vi "Get Window Constants.vi"(11 "window info":T1={"window type"=10, "window length"=2048} {"window type" items=["None"=0, "Hanning"=1, "Hamming"=2, "Blackman-Harris"=3, "Exact Blackman"=4, "Blackman"=5, "Flat Top"=6, "4 Term B-Harris"=7, "7 Term B-Harris"=8, "Low Sidelobe"=9, "Gaussian"=62]; "window length" min=0}) -> (1 "multiply factor":dbl format="%.2f", 3 "window constants":cluster{"eq noise BW":dbl, "coherent gain":dbl} {"coherent gain" format="%.2f"; "eq noise BW" format="%.2f"})   [LabVIEW 2017, in "SoundVib_Gabor.lvlib"]
uses:
  <vilib>/addons/Sound and Vibration/Order Analysis/Gabor Order Tracking/SoundVib_Gabor.lvlib
  <vilib>/addons/Sound and Vibration/Order Analysis/Ref Gabor Order Tracking/window information.ctl
  <vilib>/Analysis/0measdsp.llb/Scaled Time Domain Window (DBL).vi
  <vilib>/Analysis/NI_AALPro.lvlib
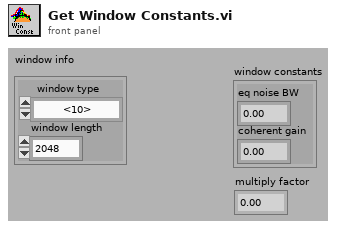
[diagram p1: front panel]
types:
  T1 = typedef "SoundVib_Gabor.lvlib/window information.ctl" = cluster{"window type":u32, "window length":i32}
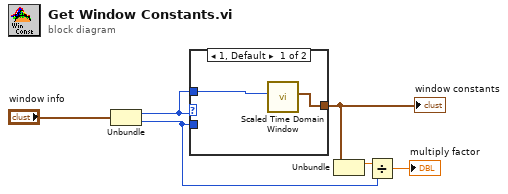
[diagram p0: block diagram]
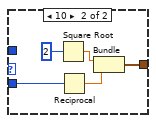
[diagram p2: hidden frame]
diagram:
  n1 = Unbundle("window info") -> ("window type"=w1:u32, "window length"=w3:i32)
  n2 = case shown="1, Default" w1 {
    tunnel: w3 -> [_ w13]
    tunnel: [w8 w9] -> w4
    tunnel: w1 -> [w7 _]
    frame 1, Default {
      n3 = call-poly <vilib>:"Scaled Time Domain Window.vi"("window"=w7) -> ("window properties"=w8:cluster{"eq noise BW":dbl, "coherent gain":dbl})  [unwired: 8 in, 2 out]
    }
    frame 10 {
      n4 = Square Root(x=2) -> (sqrt(x)=w11:dbl)
      n5 = Reciprocal(x=w13) -> (1/x=w10:dbl)
      n6 = Bundle(w11, w10) -> (w9:cluster{dbl, dbl})  [unwired: 1 in]
    }
  }
  "window constants" <- w4
  n7 = Unbundle(w4) -> ("eq noise BW"=w5:dbl)  [unwired: 1 out]
  n8 = Divide(x=w5, y=w3) -> (x/y=→"multiply factor":dbl)
